vi "Select Waveforms.vi"(8 "error in (no error)":errorcluster, 10 "Selector Input":bool[](array[boolean]), 11 "All Signals":waveform(dbl)[](array[waveform])) -> (0 "error out":errorcluster, 3 "Selected Signals":waveform(dbl)[](array[waveform]))   [LabVIEW 2013]
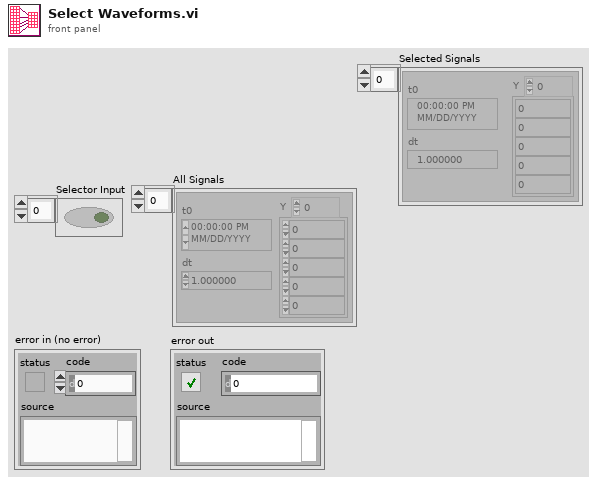
[diagram p1: front panel]
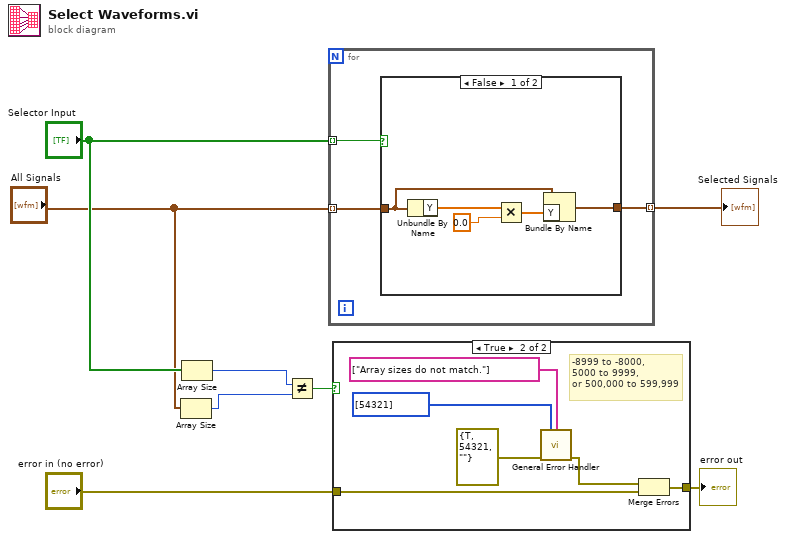
[diagram p0: block diagram]
diagram:
  n1 = Array Size(array="All Signals") -> (size(s)=w3:i32)
  n2 = Array Size(array="Selector Input") -> (size(s)=w7:i32)
  n3 = Not Equal?(x=w7, y=w3) -> (x != y?=w6:bool)
  n4 = for {
    tunnel: "All Signals" -> [w10] mode=indexing
    tunnel: "Selector Input" -> [w11] mode=indexing
    tunnel: [w9] -> w1 mode=indexing
    n5 = case shown="False" w11 {
      tunnel: w10 -> [w13 w17]
      tunnel: [w14 w17] -> w9
      frame False {
        n6 = Unbundle By Name(w13) -> ("Y"=w16:dbl[])
        n7 = Multiply(x=w16, y=0.0) -> (x*y=w12:dbl[])
        n8 = Bundle By Name(cluster=w13, "Y"=w12) -> (w14:waveform(dbl))
      }
      frame True {
      }
    }
  }
  "Selected Signals" <- w1
  n9 = case shown="True" w6 {
    tunnel: "error in (no error)" -> [w18 w20]
    tunnel: [w18 w21] -> w4
    frame False {
    }
    frame True {
      # "-8999 to -8000,\n5000 to 9999,\nor 500,000 to 599,999"
      n10 = call <vilib>:"General Error Handler.vi"("[user-defined codes]"=i32[] [54321], "[user-defined descriptions]"=string[] ["Array sizes do not match."], "error in (no error)"=errorcluster {"status"=TRUE, "code"=54321, "source"=""}) -> ("error out"=w19:errorcluster)  [unwired: 8 in, 4 out]
      n11 = Merge Errors(w19, w20) -> (w21:errorcluster)
    }
  }
  "error out" <- w4
